vi "剖面多参数上传.vi"(11 "错误输入（无错误）":errorcluster) -> (15 "error out":errorcluster)   [LabVIEW 2016, in "数据传输系统-03.lvlib"]
uses:
  <vilib>/Utility/config.llb/Write Key (String).vi
  <vilib>/Utility/config.llb/Read Key (String).vi
  <vilib>/Utility/config.llb/NI_LVConfig.lvlib
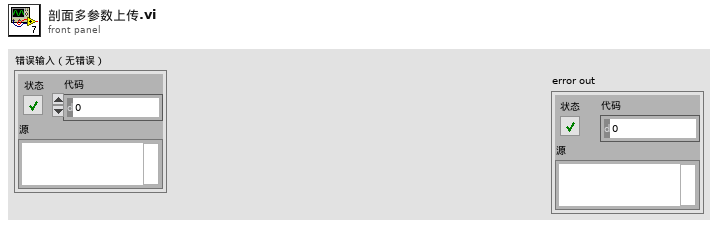
[diagram p1: front panel]
types:
  T1 = cluster{"setini":string, "sysini":string, "hechaini":string, "actualwrite":string, "actualread":string, "datasent":string, "反控命令信息队列":string, "反控与仪器交互":string}
  T2 = typedef "NI_LVConfig.lvlib/Config Data RefNum.ctl" = refnum<k1>
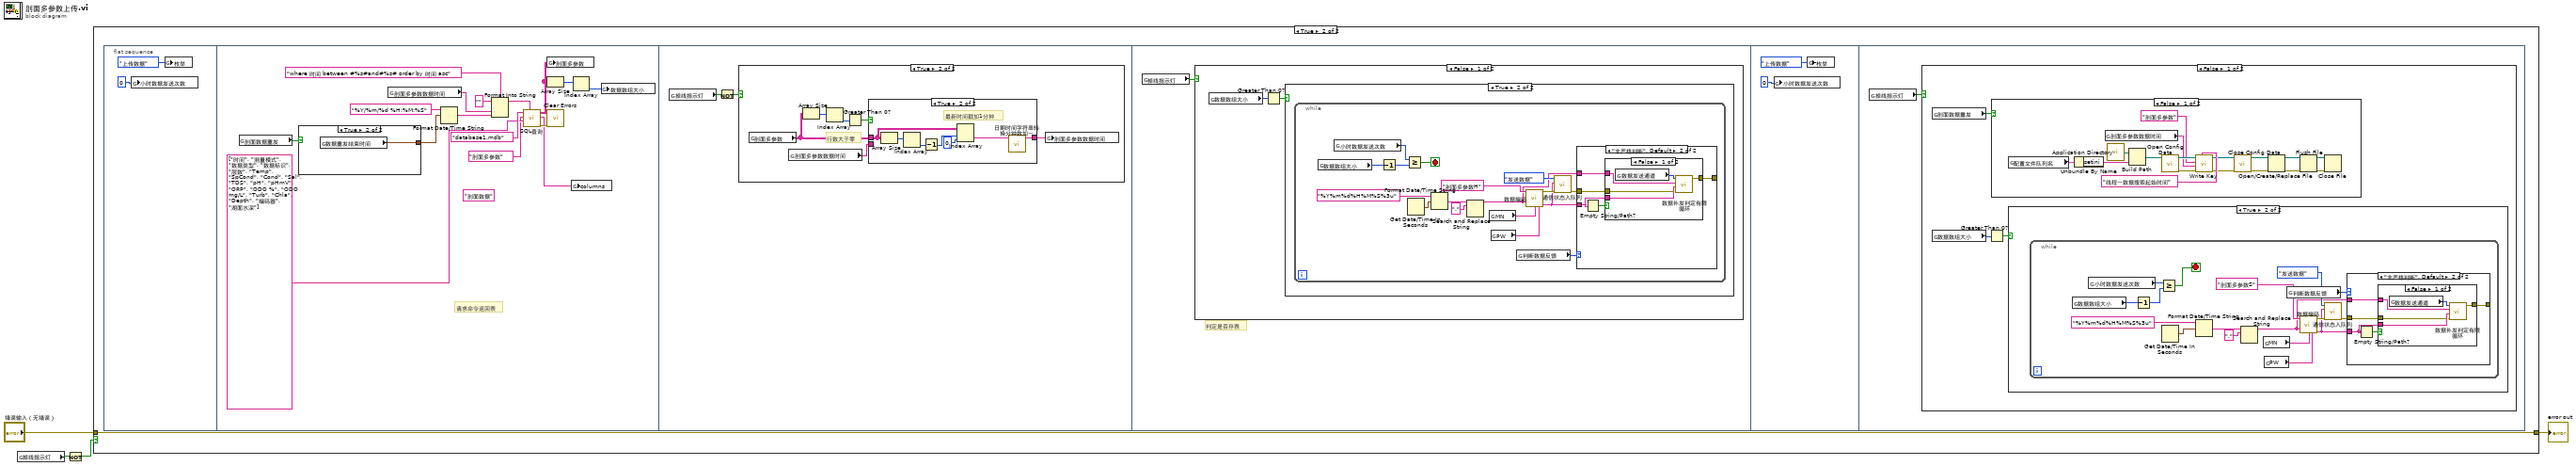
[diagram p0: block diagram]
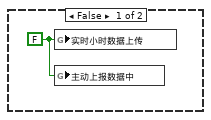
[diagram p2: hidden frame]
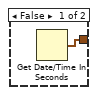
[diagram p3: hidden frame]
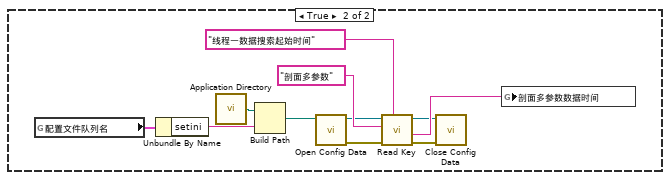
[diagram p10: hidden frame]
diagram:
  n1 = global read "全局 数据发送重叠.vi" "掉线指示灯"() -> (w4:bool)
  n2 = Not(x=w4) -> (.not. x?=w1:bool)
  n3 = case shown="True" w1 {
    tunnel: [_ w6] -> w3
    tunnel: "错误输入（无错误）" -> [_ w6]
    frame False {
      w5 = FALSE ("小时数据上传")
      n4 = global write "全局1.vi" "实时小时数据上传"(w5) -> ()
      n5 = global write "全局 数据发送重叠.vi" "主动上报数据中"(w5) -> ()
    }
    frame True {
      n6 = flat-sequence {
        frame #0 {
          n7 = global write "全局 小时数据发送次数.vi" "小时数据发送次数"(0 ("小时数据发送次数")) -> ()
          n8 = global write "全局1.vi" "枚举"(enum16{"返回请求应答", "上传数据", "返回执行结果"}."上传数据" ("枚举")) -> ()
        }
        frame #1 {
          (unwired) "剖面数据"
          # "请求命令返回表"
          n9 = global read "断电保存全局.vi" "剖面数据重发"() -> (w13:bool)
          n10 = case shown="True" w13 {
            tunnel: [w25 w26] -> w12
            frame False {
              n11 = Get Date/Time In Seconds() -> (seconds since 1Jan1904=w25:timestamp)
            }
            frame True {
              n12 = global read "断电保存全局.vi" "数据重发结束时间"() -> (w26:timestamp)
            }
          }
          n13 = global read "全局 水样时间.vi" "剖面多参数数据时间"() -> (w20:string)
          n14 = Format Date/Time String(time format string (%c)="%Y/%m/%d %H:%M:%S" ("时间格式字符串(%c)"), seconds (now)=w12) -> (date/time string=w19:string)  [unwired: 1 in]
          n15 = Format Into String(format string="where 时间 between #%s#and#%s# order by 时间 asc" ("condition"), initial string="" ("初始字符串"), w20, w19) -> (resulting string=w18:string)  [unwired: 1 in, 1 out]
          n16 = call "SQL查询.vi"("condition"=w18, "columns"=string[] ["时间", "测量模式", "数据类型", "数据标识", "层数", "Temp", "SpCond", "Cond", "Sal", "TDS", "pH", "pHmV", "ORP", "ODO %", "ODO mg/L", "Turb", "Chla", "Depth", "编码器", "湖面水深"] ("columns 2"), "table输入"="剖面多参数", "database"="database1.mdb") -> ("error out"=w14:errorcluster, "columns输出"=w11:string[], "data"=w17:string[][])  [unwired: 4 in, 1 out]
          n17 = global write "全局 所有参数.vi" "剖面多参数"(w17) -> ()
          n18 = Array Size(array=w17) -> (size(s)=w16:i32[])
          n19 = call <vilib>:"Clear Errors.vi"("error in (no error)"=w14) -> ()  [unwired: 5 in, 2 out]
          n20 = global write "全局 所有参数.vi" "columns"(w11) -> ()
          n21 = Index Array(array=w16) -> (element=w15:i32)  [unwired: 1 in]
          n22 = global write "全局 数据数组大小.vi" "数据数组大小"(w15) -> ()
        }
        frame #2 {
          n23 = global read "全局 数据发送重叠.vi" "掉线指示灯"() -> (w28:bool)
          n24 = Not(x=w28) -> (.not. x?=w27:bool)
          n25 = case shown="True" w27 {
            frame False {
            }
            frame True {
              # "行数大于零"
              n26 = global read "全局 所有参数.vi" "剖面多参数"() -> (w33:string[][])
              n27 = global read "全局 水样时间.vi" "剖面多参数数据时间"() -> (w34:string)
              n28 = Array Size(array=w33) -> (size(s)=w30:i32[])
              n29 = Index Array(array=w30) -> (element=w31:i32)  [unwired: 1 in]
              n30 = Greater Than 0?(x=w31) -> (x > 0?=w32:bool)
              n31 = case shown="True" w32 {
                tunnel: w33 -> [_ w39]
                tunnel: [w35 w36] -> w29
                tunnel: w34 -> [w35 _]
                frame False {
                }
                frame True {
                  # "最新时间戳加1分钟"
                  n32 = Array Size(array=w39) -> (size(s)=w41:i32[])
                  n33 = Index Array(array=w41) -> (element=w40:i32)  [unwired: 1 in]
                  n34 = Decrement(x=w40) -> (x-1=w38:i32)
                  n35 = Index Array(array=w39, index (row)=w38, index (col)=0 ("禁用的索引 (列)")) -> (element=w42:string)
                  n36 = call "日期时间字符串转换分钟数加一.vi"("data[0]"=w42) -> ("日期/时间字符串"=w36:string)  [unwired: 10 in]
                }
              }
              n37 = global write "全局 水样时间.vi" "剖面多参数数据时间"(w29) -> ()
            }
          }
        }
        frame #3 {
          # "判定是否存表"
          n38 = global read "全局 数据发送重叠.vi" "掉线指示灯"() -> (w43:bool)
          n39 = case shown="False" w43 {
            frame False {
              n40 = global read "全局 数据数组大小.vi" "数据数组大小"() -> (w44:i32)
              n41 = Greater Than 0?(x=w44) -> (x > 0?=w45:bool)
              n42 = case shown="True" w45 {
                frame False {
                }
                frame True {
                  n43 = while {
                    stop <- w51 stop-if-true
                    n44 = global read "全局 数据数组大小.vi" "数据数组大小"() -> (w53:i32)
                    n45 = global read "全局 小时数据发送次数.vi" "小时数据发送次数"() -> (w54:i32)
                    n46 = Decrement(x=w53) -> (x-1=w52:i32)
                    n47 = Greater Or Equal?(x=w54, y=w52) -> (x >= y?=w51:bool)
                    n48 = Get Date/Time In Seconds() -> (seconds since 1Jan1904=w60:timestamp)
                    n49 = Format Date/Time String(time format string (%c)="%Y%m%d%H%M%S%3u" ("时间格式字符串(%c)"), seconds (now)=w60) -> (date/time string=w59:string)  [unwired: 1 in]
                    n50 = Search and Replace String(input string=w59, search string="." ("搜索字符串")) -> (result string=w48:string)  [unwired: 6 in, 3 out]
                    n51 = global read "断电保存全局.vi" "MN"() -> (w57:string)
                    n52 = global read "断电保存全局.vi" "PW"() -> (w56:string)
                    n53 = global read "断电保存全局.vi" "判断数据反馈"() -> (w49:enum16{"非严格判断", "严格判断", "不判断"})
                    n54 = call "数据编码.vi"("table输入"="剖面多参数H" ("新元素/子数组"), "QN"=w48, "MN"=w57, "PW"=w56) -> ("错误常量"=w55:errorcluster, "通讯包字符串"=w47:string)  [unwired: 10 in]
                    n55 = call "通信状态入队列.vi"("错误输入（无错误）"=w55, "发送报文"=w47, "枚举"=enum16{"打开连接", "发送数据", "读取数据", "数据处理", "关闭连接"}."发送数据") -> ("错误输出"=w46:errorcluster)  [unwired: 8 in]
                    n56 = case shown="\"非严格判断\", Default" w49 {
                      tunnel: [_ w67] -> _
                      tunnel: w47 -> [_ w66]
                      tunnel: w48 -> [_ w65]
                      tunnel: w46 -> [_ w63]
                      frame "不判断" {
                      }
                      frame "非严格判断", Default {
                        n57 = Empty String/Path?(string/path=w66) -> (empty?=w64:bool)
                        n58 = case shown="False" w64 {
                          tunnel: [w72 _] -> w67
                          tunnel: w66 -> [w71 _]
                          tunnel: w65 -> [w69 _]
                          tunnel: w63 -> [w68 _]
                          frame False {
                            n59 = global read "断电保存全局.vi" "数据发送通道"() -> (w70:enum16{"TCP", "VISA"})
                            n60 = call "数据补发判定有限循环.vi"("错误输入（无错误）"=w68, "数据输入"=w71, "QN"=w69, "数据发送通道"=w70) -> ("error out"=w72:errorcluster)  [unwired: 7 in]
                          }
                          frame True {
                          }
                        }
                      }
                    }
                  }
                }
              }
            }
            frame True {
            }
          }
        }
        frame #4 {
          n61 = global write "全局 小时数据发送次数.vi" "小时数据发送次数"(0 ("小时数据发送次数")) -> ()
          n62 = global write "全局1.vi" "枚举"(enum16{"返回请求应答", "上传数据", "返回执行结果"}."上传数据" ("枚举")) -> ()
        }
        frame #5 {
          n63 = global read "全局 数据发送重叠.vi" "掉线指示灯"() -> (w75:bool)
          n64 = case shown="False" w75 {
            frame False {
              n65 = global read "断电保存全局.vi" "剖面数据重发"() -> (w76:bool)
              n66 = global read "全局 数据数组大小.vi" "数据数组大小"() -> (w78:i32)
              n67 = Greater Than 0?(x=w78) -> (x > 0?=w77:bool)
              n68 = case shown="False" w76 {
                frame False {
                  n69 = global read "全局1.vi" "配置文件队列名"() -> (w79:T1)
                  n70 = Unbundle By Name(w79) -> ("setini"=w80:string)
                  n71 = global read "全局 水样时间.vi" "剖面多参数数据时间"() -> (w81:string)
                  n72 = call <vilib>:"Application Directory.vi"() -> ("Application Directory"=w89:path)
                  n73 = Build Path(base path=w89, name or relative path=w80) -> (appended path=w90:path)
                  n74 = call <vilib>:"Open Config Data.vi"("configuration file path"=w90) -> ("error out"=w92:errorcluster, "refnum"=w91:T2)  [unwired: 8 in, 1 out]
                  n75 = call-poly <vilib>:"Write Key.vi"("section"="线程一数据搜索起始时间", "error in (no error)"=w92, "value"=w81, "key"="剖面多参数", "refnum"=w91) -> ("error out"=w94:errorcluster, "refnum out"=w93:T2)  [unwired: 4 in, 1 out]
                  n76 = call <vilib>:"Close Config Data.vi"("error in (no error)"=w94, "refnum"=w93) -> ("error out"=w82:errorcluster, "file path"=w83:path)  [unwired: 8 in]
                  n77 = Open/Create/Replace File(file path (use dialog)=w83, error in=w82) -> (refnum out=w85:refnum<file>, error out=w84:errorcluster)  [unwired: 4 in, 1 out]
                  n78 = Flush File(refnum=w85, error in=w84) -> (refnum out=w86:refnum<file>, error out=w87:errorcluster)
                  n79 = Close File(refnum=w86, error in=w87) -> ()  [unwired: 2 out]
                }
                frame True {
                  n80 = global read "全局1.vi" "配置文件队列名"() -> (w96:T1)
                  n81 = Unbundle By Name(w96) -> ("setini"=w103:string)
                  n82 = call <vilib>:"Application Directory.vi"() -> ("Application Directory"=w102:path)
                  n83 = Build Path(base path=w102, name or relative path=w103) -> (appended path=w104:path)
                  n84 = call <vilib>:"Open Config Data.vi"("configuration file path"=w104) -> ("error out"=w99:errorcluster, "refnum"=w98:T2)  [unwired: 8 in, 1 out]
                  n85 = call-poly <vilib>:"Read Key.vi"("section"="线程一数据搜索起始时间", "error in (no error)"=w99, "key"="剖面多参数", "refnum"=w98) -> ("error out"=w101:errorcluster, "value"=w106:string, "refnum out"=w100:T2)  [unwired: 4 in, 1 out]
                  n86 = call <vilib>:"Close Config Data.vi"("error in (no error)"=w101, "refnum"=w100) -> ()  [unwired: 8 in, 2 out]
                  n87 = global write "全局 水样时间.vi" "剖面多参数数据时间"(w106) -> ()
                }
              }
              n88 = case shown="True" w77 {
                frame False {
                }
                frame True {
                  n89 = while {
                    stop <- w112 stop-if-true
                    n90 = global read "全局 数据数组大小.vi" "数据数组大小"() -> (w114:i32)
                    n91 = global read "全局 小时数据发送次数.vi" "小时数据发送次数"() -> (w115:i32)
                    n92 = Decrement(x=w114) -> (x-1=w113:i32)
                    n93 = Greater Or Equal?(x=w115, y=w113) -> (x >= y?=w112:bool)
                    n94 = Get Date/Time In Seconds() -> (seconds since 1Jan1904=w121:timestamp)
                    n95 = Format Date/Time String(time format string (%c)="%Y%m%d%H%M%S%3u" ("时间格式字符串(%c)"), seconds (now)=w121) -> (date/time string=w120:string)  [unwired: 1 in]
                    n96 = Search and Replace String(input string=w120, search string="." ("搜索字符串")) -> (result string=w109:string)  [unwired: 6 in, 3 out]
                    n97 = global read "断电保存全局.vi" "MN"() -> (w118:string)
                    n98 = global read "断电保存全局.vi" "PW"() -> (w117:string)
                    n99 = global read "断电保存全局.vi" "判断数据反馈"() -> (w110:enum16{"非严格判断", "严格判断", "不判断"})
                    n100 = call "数据编码.vi"("table输入"="剖面多参数S" ("新元素/子数组"), "QN"=w109, "MN"=w118, "PW"=w117) -> ("错误常量"=w116:errorcluster, "通讯包字符串"=w108:string)  [unwired: 10 in]
                    n101 = call "通信状态入队列.vi"("错误输入（无错误）"=w116, "发送报文"=w108, "枚举"=enum16{"打开连接", "发送数据", "读取数据", "数据处理", "关闭连接"}."发送数据") -> ("错误输出"=w107:errorcluster)  [unwired: 8 in]
                    n102 = case shown="\"非严格判断\", Default" w110 {
                      tunnel: [_ w128] -> _
                      tunnel: w108 -> [_ w127]
                      tunnel: w109 -> [_ w126]
                      tunnel: w107 -> [_ w124]
                      frame "不判断" {
                      }
                      frame "非严格判断", Default {
                        n103 = Empty String/Path?(string/path=w127) -> (empty?=w125:bool)
                        n104 = case shown="False" w125 {
                          tunnel: [w133 _] -> w128
                          tunnel: w127 -> [w132 _]
                          tunnel: w126 -> [w130 _]
                          tunnel: w124 -> [w129 _]
                          frame False {
                            n105 = global read "断电保存全局.vi" "数据发送通道"() -> (w131:enum16{"TCP", "VISA"})
                            n106 = call "数据补发判定有限循环.vi"("错误输入（无错误）"=w129, "数据输入"=w132, "QN"=w130, "数据发送通道"=w131) -> ("error out"=w133:errorcluster)  [unwired: 7 in]
                          }
                          frame True {
                          }
                        }
                      }
                    }
                  }
                }
              }
            }
            frame True {
            }
          }
        }
      }
    }
  }
  "error out" <- w3
